vi "Close Document.vi"(0 "object in":refnum<class "Document.lvclass">, 5 "error in (no error)":errorcluster) -> (14 "object out":refnum<class "Document.lvclass">, 19 "error out":errorcluster)   [LabVIEW 2014, in "Document.lvclass"]
uses:
  Document.lvclass
  Document.lvclass/Document.ctl
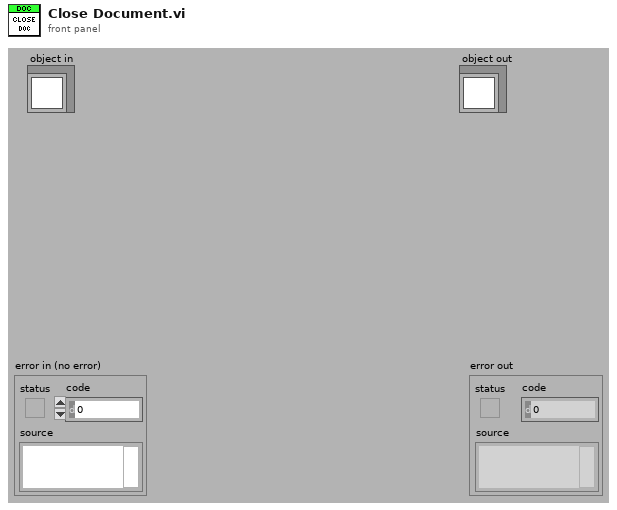
[diagram p1: front panel]
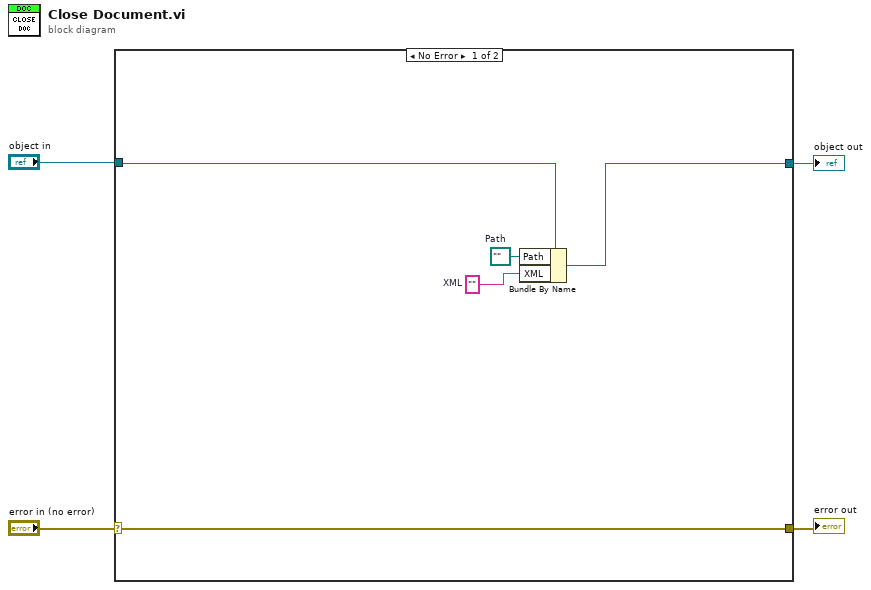
[diagram p0: block diagram]
diagram:
  n1 = case shown="No Error" "error in (no error)" {
    selector: "error in (no error)" -> [w9 w11]
    tunnel: [w9 w11] -> w3
    tunnel: [w7 w10] -> w1
    tunnel: "object in" -> [w8 w10]
    frame No Error {
      w5 = ""  # XML
      w6 = path ""  # Path
      n2 = Bundle By Name(cluster=w8, "Path"=w6, "XML"=w5) -> (w7:refnum<class "Document.lvclass">)
    }
    frame Error {
    }
  }
  "error out" <- w3
  "object out" <- w1
